vi "ADAM 5000 Get Temperatures.vi"(11 "Remote IP Address 2":string="192.168.11.50") -> (1 "TC String Array":string[](array[string]), 2 "TC Array":dbl[](array[numeric])=[195.33139999999997, 1369.6815, 1369.6815, 1369.6815, 1369.6815, 1369.6815, 1369.6815])   [LabVIEW 2016]
uses:
  nimodbus121/71/vi.lib/NI Modbus.llb/MB Modbus Command.ctl
panel:
  out "error out":errorcluster
  in  "Modbus Command":T1={"Function Code"=3, "Starting Address"=16, "Quantity"=7, "Data"=[], "Discrete"=[]} {"Function Code" items=["Read Coils"=1, "Read Discrete Inputs"=2, "Read Holding Registers"=3, "Read Input Registers"=4, "Write Single Coil"=5, "Write Single Register"=6, "Read Exception Status"=7, "Write Multiple Coils"=15, "Write Multiple Registers"=16]}
  out "Slave Input Registers 2":u16[](array[numeric])=[9346, 65535, 65535, 65535, 65535, 65535, 65535] caption="Slave Input Registers (Read Only)"
  in  "Remote Port 2":u16=502
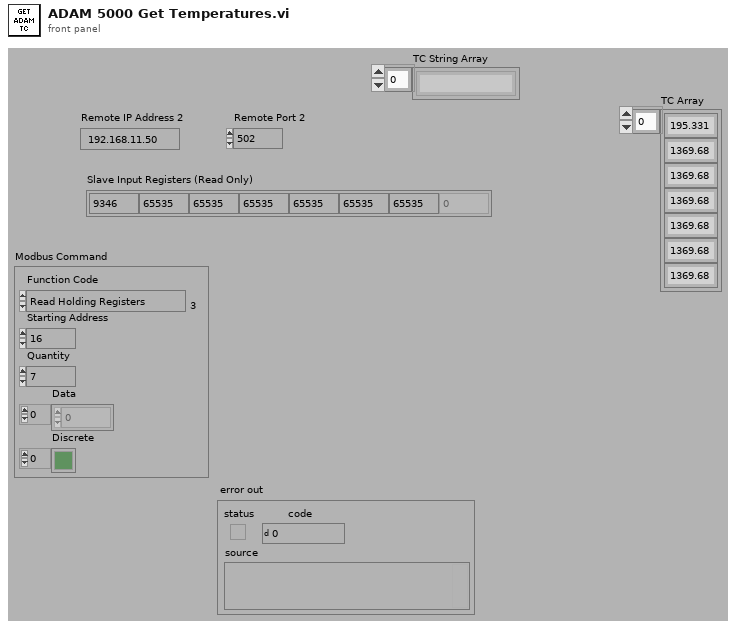
[diagram p1: front panel]
types:
  T1 = typedef "MB Modbus Command.ctl" = cluster{"Function Code":u8, "Starting Address":u16, "Quantity":u16, "Data":u16[], "Discrete":bool[]}
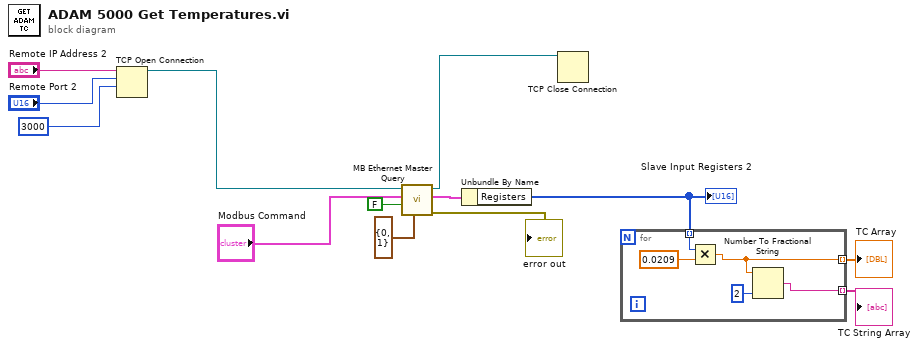
[diagram p0: block diagram]
diagram:
  n1 = TCP Open Connection(address="Remote IP Address 2", remote port or service name="Remote Port 2", timeout ms (60000)=3000) -> (connection ID=w11:refnum<k5>)  [unwired: 2 in, 1 out]
  n2 = call "MB Ethernet Master Query.vi"("MBAP Header"=cluster{"Transaction ID":u16, "Unit ID":u8} {"Transaction ID"=0, "Unit ID"=1}, "Use MODBUS Data Unit?"=FALSE, "Modbus Command"="Modbus Command", "TCP Connection Refnum in"=w11) -> ("error out"=→"error out":errorcluster, "Registers"=w7:cluster{"Registers":u16[], "Discrete":bool[]}, "TCP Connection Refnum (dup)"=w10:refnum<k5>)  [unwired: 3 in, 2 out]
  n3 = Unbundle By Name(w7) -> ("Registers"=w3:u16[])
  "Slave Input Registers 2" <- w3
  n4 = TCP Close Connection(connection ID=w10) -> ()  [unwired: 2 in, 2 out]
  n5 = for {
    tunnel: w3 -> [w18] mode=indexing
    tunnel: [w16] -> w2 mode=indexing
    tunnel: [w14] -> w1 mode=indexing
    n6 = Multiply(x=w18, y=0.0209) -> (x*y=w16:dbl)
    n7 = Number To Fractional String(number=w16, precision (6)=i16 2) -> (F-format string=w14:string)  [unwired: 2 in]
  }
  "TC Array" <- w2
  "TC String Array" <- w1
